vi "InsertImageNoMaskGreyscale.vi"(7 "Offset (Default: 0,0)":T1, 8 "error in (no error)":errorcluster, 9 "Greyscale Image Destination":refnum<data-value>, 10 "Greyscale Image Child":refnum<data-value>, 11 "Greyscale Image Parent":refnum<data-value>) -> (0 "error out":errorcluster, 3 "Greyscale Image Destination (duplicate)":refnum<data-value>)   [LabVIEW 2020, in "g_ar_toolkit.image.lvlib"]
uses:
  g_ar_toolkit.image.lvlib
  g_ar_toolkit.common/Image Point (Integer).ctl
  <vilib>/Utility/error.llb/Error Cluster From Error Code.vi
  5e3288c8-ee88-4cfe-89cf-31ceca475f5a.vi
  g_ar_toolkit.common/g_ar_toolkit.common.lvlib
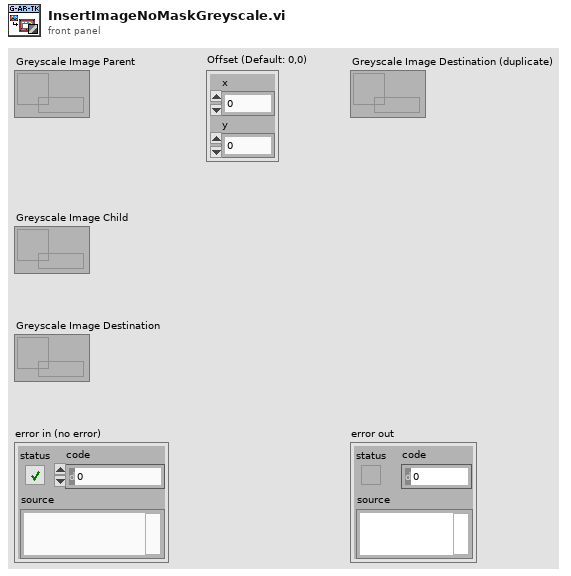
[diagram p1: front panel]
types:
  T1 = typedef "g_ar_toolkit.common.lvlib/Image Point (Integer).ctl" = cluster{"x":i32, "y":i32}
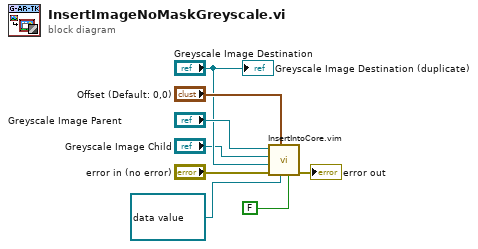
[diagram p0: block diagram]
diagram:
  n1 = call "InsertIntoCore.vim"("Has Mask"=FALSE, "Mask"=refnum<data-value> refnum, "Offset"="Offset (Default: 0,0)", "error in (no error)"="error in (no error)", "Dst"="Greyscale Image Destination", "Src_Child"="Greyscale Image Child", "Src_Parent"="Greyscale Image Parent") -> ("error out"=→"error out":errorcluster)  [unwired: 4 in]
  "Greyscale Image Destination (duplicate)" <- "Greyscale Image Destination"
